vi "Sonderzeichen auswerten.vi"(11 "String":string) -> (2 "Anzahl":i32, 3 "Suchstring":string)   [LabVIEW 2015, in "Sprachverwaltung.lvlib"]
uses:
  Sprachverwaltung.lvlib
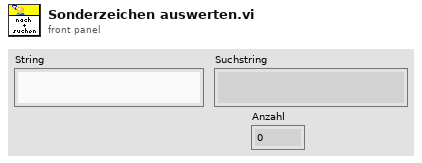
[diagram p1: front panel]
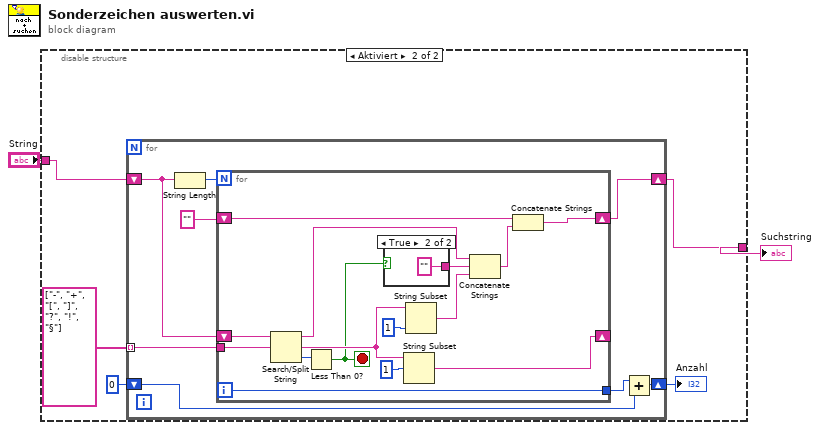
[diagram p0: block diagram]
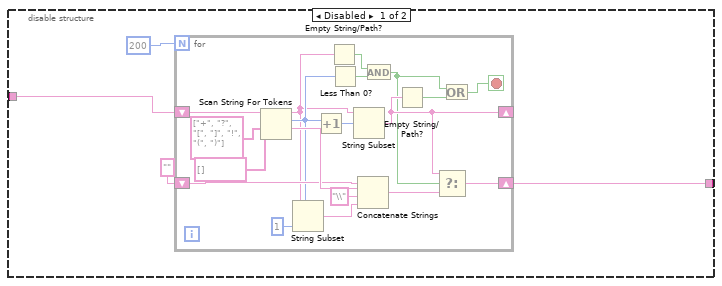
[diagram p2: hidden frame]
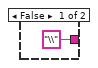
[diagram p3: hidden frame]
diagram:
  n1 = disable-structure shown="Aktiviert" {
    disable-tunnel: "String" -> [w4 w29]
    disable-tunnel: [w3 w28] -> w1
    frame Disabled {
      n2 = for {
        N: 200 -> [_]
        shift-right: [w11] -> _
        shift-left: w4 -> [w25]
        shift-right: [w12] -> w3
        shift-left: "" -> [w19]
        stop <- w14 stop-if-true
        n3 = Scan String For Tokens(6:string[] [] ("Trennzeichen (\\s,\\t,\\r,\\n)"), 7:string[] ["+", "?", "[", "]", "!", "(", ")"] ("Operatoren (keine)"), 9:w25) -> (1:w24:string, 2:w16:i32, 3:w10:string)  [unwired: 3 in, 1 out]
        n4 = String Subset(string=w10, offset (0)=w16, length (rest)=1 ("Länge (Rest)")) -> (substring=w20:string)
        n5 = Increment(x=w16) -> (x+1=w18:i32)
        n6 = Empty String/Path?(string/path=w10) -> (empty?=w8:bool)
        n7 = Less Than 0?(x=w16) -> (x < 0?=w9:bool)
        n8 = String Subset(string=w10, offset (0)=w18) -> (substring=w11:string)  [unwired: 1 in]
        n9 = Concatenate Strings(w19, w24, "\\" ("String"), w20) -> (w13:string)
        n10 = And(x=w8, y=w9) -> (x .and. y?=w7:bool)
        n11 = Empty String/Path?(string/path=w11) -> (empty?=w15:bool)
        n12 = Select(t=w11, s=w7, f=w13) -> (s? t:f=w12:string)
        n13 = Or(x=w7, y=w15) -> (x .or. y?=w14:bool)
      }
    }
    frame Enabled {
      n14 = for {
        tunnel: string[] ["-", "+", "[", "]", "?", "!", "§"] -> [w36] mode=indexing
        shift-right: [w34] -> w28
        shift-left: w29 -> [w37]
        shift-right: [w31] -> w26
        shift-left: 0 -> [w32]
        n15 = String Length(string=w37) -> (length=w38:i32)
        n16 = for {
          N: w38 -> [_]
          shift-right: [w51] -> w34
          shift-left: "" -> [w52]
          shift-right: [w43] -> _
          shift-left: w37 -> [w53]
          tunnel: w36 -> [w40]
          tunnel: [w39] -> w33
          i -> [w39]
          stop <- w41 stop-if-true
          n17 = Search/Split String(string=w53, search string/char (-)=w40) -> (substring before match=w50:string, match + rest of string=w44:string, offset of match=w42:i32)  [unwired: 1 in]
          n18 = Less Than 0?(x=w42) -> (x < 0?=w41:bool)
          n19 = case shown="True" w41 {
            tunnel: ["\\" ("String") "" ("String")] -> w49
            frame False {
            }
            frame True {
            }
          }
          n20 = String Subset(string=w44, offset (0)=1 ("Länge (Rest)")) -> (substring=w43:string)  [unwired: 1 in]
          n21 = String Subset(string=w44, length (rest)=1 ("Länge (Rest)")) -> (substring=w46:string)  [unwired: 1 in]
          n22 = Concatenate Strings(w50, w49, w46) -> (w48:string)
          n23 = Concatenate Strings(w52, w48) -> (w51:string)
        }
        n24 = Add(x=w33, y=w32) -> (x+y=w31:i32)
      }
      "Anzahl" <- w26
    }
  }
  "Suchstring" <- w1
